vi "Write Prev SET parameters.vi"(8 "error in (no error)":errorcluster, 10 "Prev SET parameters":T1, 11 "Simulated_CCD_Camera in":refnum<class "Simulated Camera.lvclass">) -> (0 "error out":errorcluster, 3 "Simulated_CCD_Camera out":refnum<class "Simulated Camera.lvclass">)   [LabVIEW 2018, in "Simulated Camera.lvclass"]
uses:
  Simulated Camera.lvclass
  Simulated Camera.lvclass/Simulated Camera.ctl
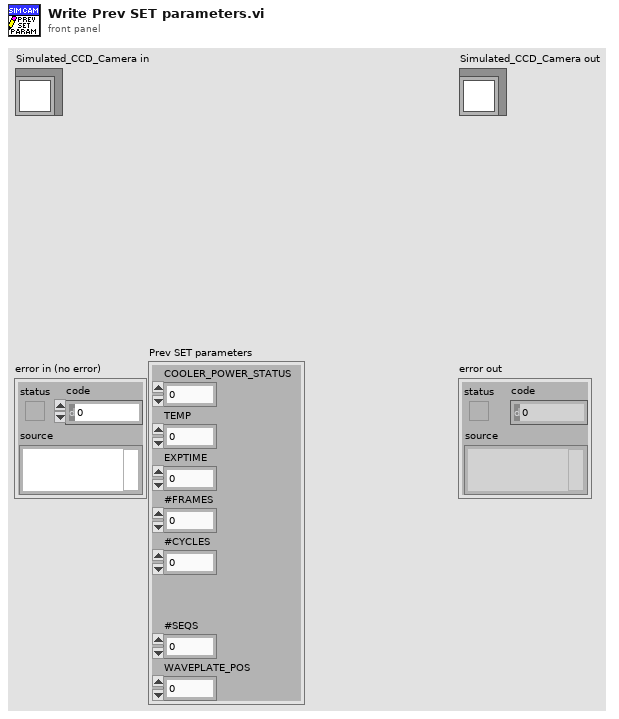
[diagram p1: front panel]
types:
  T1 = cluster{"COOLER_POWER_STATUS":u16, "TEMP":i32, "EXPTIME":dbl, "#FRAMES":u32, "#CYCLES":u32, "#SEQS":u32, "WAVEPLATE_POS":u16}
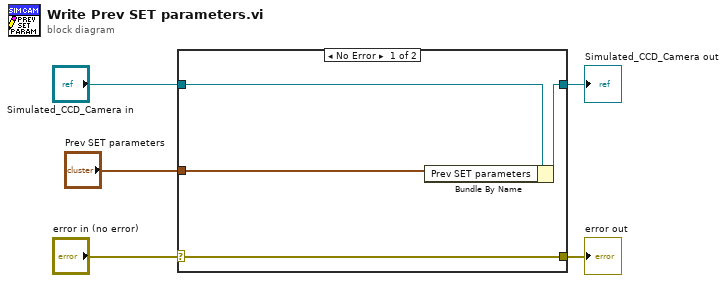
[diagram p0: block diagram]
diagram:
  n1 = case shown="No Error" "error in (no error)" {
    selector: "error in (no error)" -> [w9 w10]
    tunnel: [w9 w10] -> w4
    tunnel: [w7 w11] -> w2
    tunnel: "Simulated_CCD_Camera in" -> [w8 w11]
    tunnel: "Prev SET parameters" -> [w6 _]
    frame No Error {
      n2 = Bundle By Name(cluster=w8, "Prev SET parameters"=w6) -> (w7:refnum<class "Simulated Camera.lvclass">)
    }
    frame Error {
    }
  }
  "error out" <- w4
  "Simulated_CCD_Camera out" <- w2
